vi "Constants.vi"() -> ()   [LabVIEW 2021]
panel:
  in  "UI Cnfiguration File":path
  in  "Instruments Configuration File":path
  in  "Config Files Folder":path=path "/home/qizhen/project"
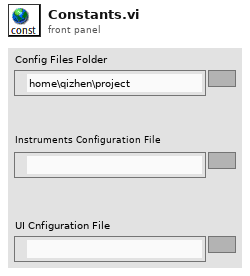
[diagram p1: front panel]
diagram:
